vi "GCS3 Read Entries.vi"(0 "Line to Parse":string, 5 "error in":errorcluster) -> (15 "Array of GCS 3.0 Block Entries":string[](array[string]), 19 "error out":errorcluster)   [LabVIEW 2020]
uses:
  Match Regular Expression.xnode
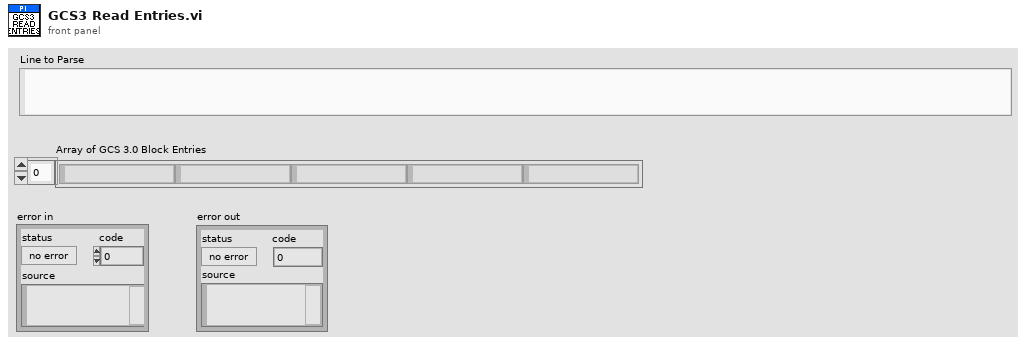
[diagram p1: front panel]
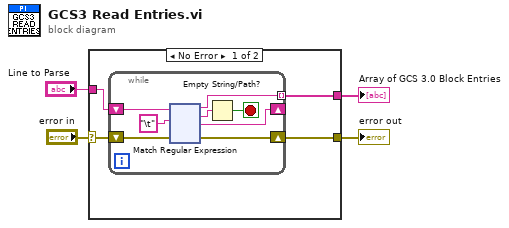
[diagram p0: block diagram]
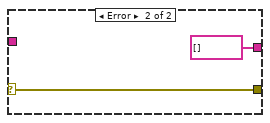
[diagram p2: hidden frame]
diagram:
  n1 = case shown="No Error" "error in" {
    selector: "error in" -> [w5 w132]
    tunnel: [w6 w132] -> w3
    tunnel: "Line to Parse" -> [w8 _]
    tunnel: [w7 string[] [] ("Array of GCS 3.0 Block Entries")] -> w1
    frame No Error {
      n2 = while {
        shift-right: [w16] -> _
        shift-left: w8 -> [w12]
        tunnel: [w15] -> w7 mode=indexing
        shift-right: [w10] -> w6
        shift-left: w5 -> [w9]
        stop <- w13 stop-if-true
        n3 = xnode "Match Regular Expression"("input string"=w12, "regular expression"="\t", "error in"=w9) -> ("before match"=w15:string, "whole match"=w14:string, "after match"=w16:string, "error out"=w10:errorcluster)  [unwired: 3 in, 1 out]
        n4 = Empty String/Path?(string/path=w14) -> (empty?=w13:bool)
      }
    }
    frame Error {
    }
  }
  "error out" <- w3
  "Array of GCS 3.0 Block Entries" <- w1
